vi "Goomba.vi"(0 "X Init":i32, 1 "Picture In":picture, 2 "Y Init":i32, 3 "Left Bound":i32=400, 4 "Dir In":T1, 5 "Right Bound":i32=775) -> (6 "Dir Out":T1, 7 "Pos Out":i32, 8 "Main Picture":picture)   [LabVIEW 2014]
uses:
  Goomba Direction.ctl
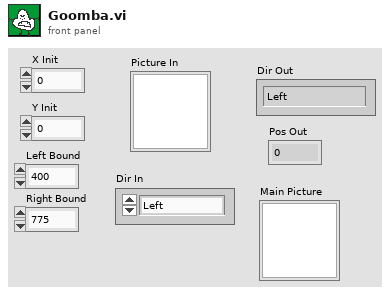
[diagram p1: front panel]
types:
  T1 = typedef "Goomba Direction.ctl" = enum16{"Left", "Right"}
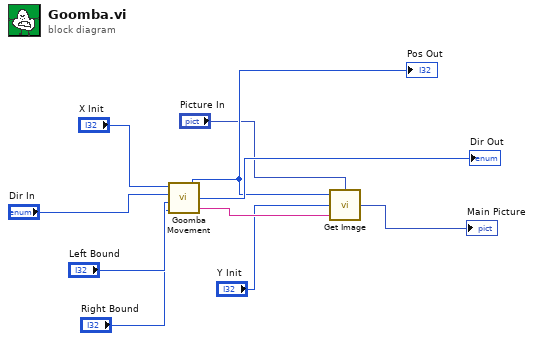
[diagram p0: block diagram]
diagram:
  n1 = call "Goomba Movement.vi"("Right Bound"="Right Bound", "Left Bound"="Left Bound", "Dir Init"="Dir In", "Pos Init"="X Init") -> ("Picture Name"=w8:string, "Dir Out"=→"Dir Out":T1, "Pos Out"=w6:i32)
  "Pos Out" <- w6
  n2 = call "Get Image.vi"("Input Picture"="Picture In", "String"=w8, "Bottom"="Y Init", "Left"=w6) -> ("Main Picture"=→"Main Picture":picture)
